vi "Read CIB.vi"(10 "COM Ref":refnum<visa-resource-name>, 11 "Cal Point":T1) -> (0 "Error Out":errorcluster, 2 "Dev Table 2":string[][](array[string]), 3 "Dev Table 1":string[][](array[string]))   [LabVIEW 2013]
uses:
  Type Defs/Cal Point Type Def.ctl
  RS485/Port Config.ctl
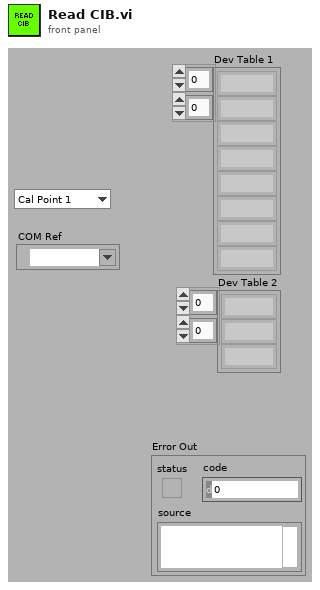
[diagram p1: front panel]
types:
  T1 = typedef "Cal Point Type Def.ctl" = enum16{"Cal Point 1", "Cal Point 2", "Cal Point 3", "Cal Point 4", "Cal Point 5", "Cal Point 6", "Cal Point 7"}
  T2 = typedef "Port Config.ctl" = cluster{"VISA resource name":refnum<visa-resource-name>, "baud rate":u32, "data bits (8)":u16, "parity (0:none)":enum16{"None", "Odd", "Even", "Mark", "Space"}, "stop bits (10: 1 bit)":u16, "flow control (0:none)":u16, "timeout (2sec)":u32}
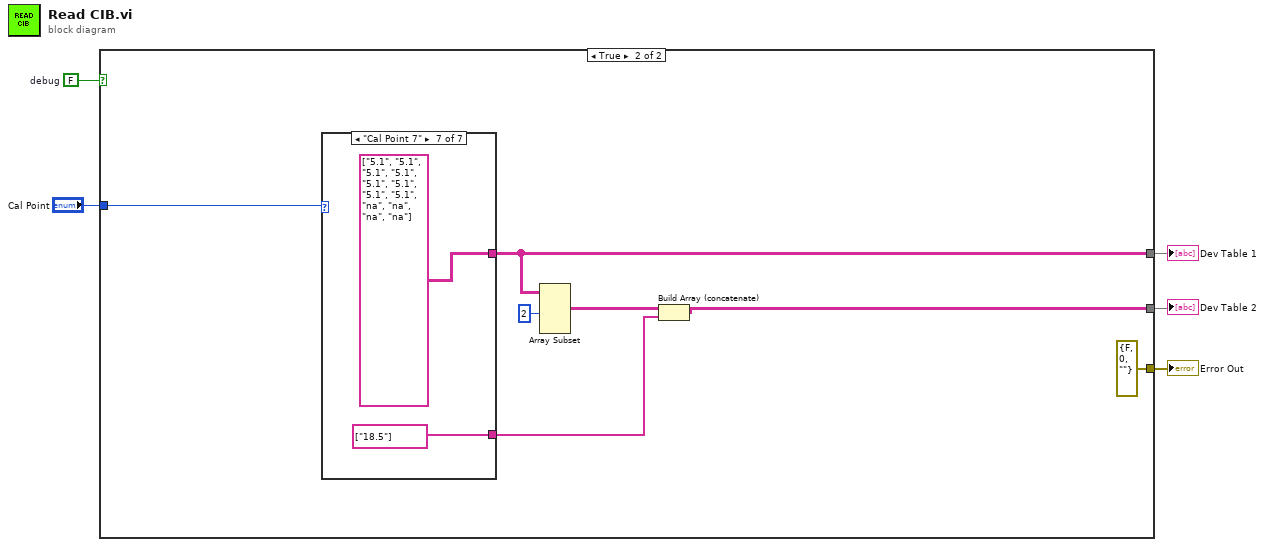
[diagram p0: block diagram]
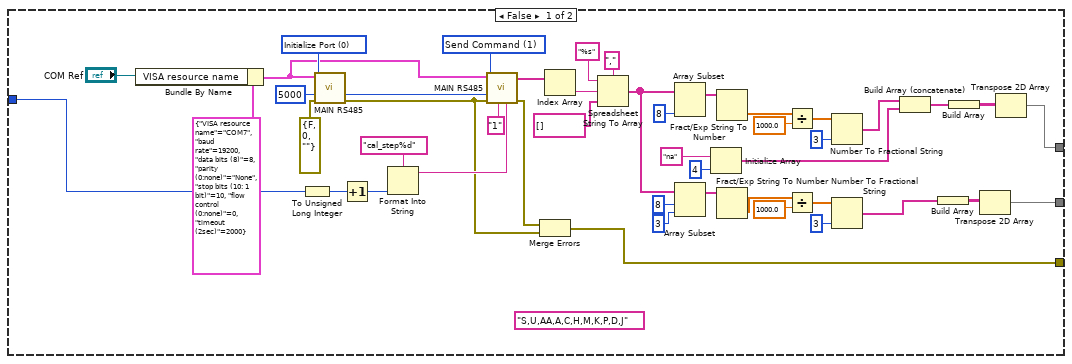
[diagram p2: hidden frame]
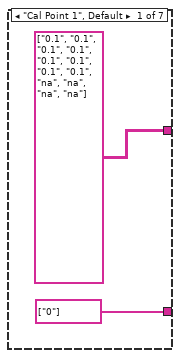
[diagram p3: hidden frame]
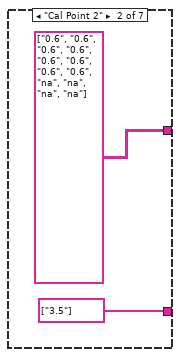
[diagram p4: hidden frame]
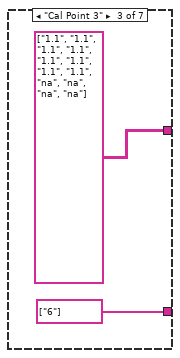
[diagram p5: hidden frame]
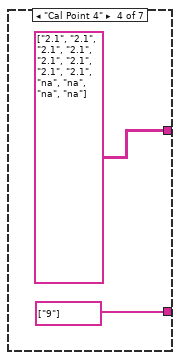
[diagram p6: hidden frame]
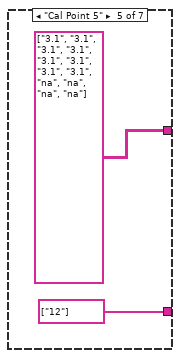
[diagram p7: hidden frame]
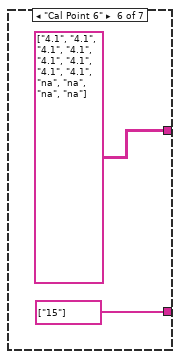
[diagram p8: hidden frame]
diagram:
  w2 = FALSE  # debug
  n1 = case shown="True" w2 {
    tunnel: "Cal Point" -> [w45 w57]
    tunnel: [w31 w56] -> w4
    tunnel: [w26 w51] -> w3
    tunnel: [w22 errorcluster {"status"=FALSE, "code"=0, "source"=""} ("Error Out")] -> w1
    frame False {
      (unwired) "S,U,AA,A,C,H,M,K,P,D,J" ("format string")
      w47 = u16 1 items=["Initialize Port", "Send Command", "Get Commands"] ("RS485 Operation")
      w18 = u32 5000 ("Timeout (ms)")
      w48 = u16 0 items=["Initialize Port", "Send Command", "Get Commands"] ("RS485 Operation")
      n2 = Bundle By Name(cluster=T2 {"VISA resource name"="COM7", "baud rate"=19200, "data bits (8)"=8, "parity (0:none)"=enum."None", "stop bits (10: 1 bit)"=10, "flow control (0:none)"=0, "timeout (2sec)"=2000} ("PortConfig"), "VISA resource name"="COM Ref") -> (w19:T2)
      n3 = To Unsigned Long Integer(number=w45) -> (unsigned 32bit integer=w44:u32)
      n4 = call "MAIN RS485.vi"("Error In"=errorcluster {"status"=FALSE, "code"=0, "source"=""}, "Timeout (ms)"=w18, "RS485 Operation"=w48, "PortConfig"=w19) -> ("Error Out"=w23:errorcluster)  [unwired: 6 in, 1 out]
      n5 = Increment(x=w44) -> (x+1=w43:u32)
      n6 = Format Into String(format string="cal_step%d" ("CIB address"), w43) -> (resulting string=w42:string)  [unwired: 2 in, 1 out]
      n7 = call "MAIN RS485.vi"("message"=w42, "CIB address"="1", "Error In"=w23, "Timeout (ms)"=w18, "RS485 Operation"=w47, "PortConfig"=w19) -> ("Error Out"=w24:errorcluster, "Return String[]"=w25:string[])  [unwired: 4 in]
      n8 = Merge Errors(w24, w23) -> (w22:errorcluster)
      n9 = Index Array(array=w25) -> (element=w20:string)  [unwired: 1 in]
      n10 = Spreadsheet String To Array(delimiter (Tab)=",", format string="%s", spreadsheet string=w20, array type (2D Dbl)=string[] []) -> (array=w29:string[])
      n11 = Array Subset(array=w29, length=8) -> (w17:string[])  [unwired: 1 in]
      n12 = Array Subset(array=w29, index=8, length=3) -> (w7:string[])
      n13 = Initialize Array("na" ("format string"), 4 ("dimension size")) -> (w34:string[])
      n14 = Fract/Exp String To Number(string=w17) -> (number=w16:dbl[])  [unwired: 3 in, 1 out]
      n15 = Fract/Exp String To Number(string=w7) -> (number=w6:dbl[])  [unwired: 3 in, 1 out]
      n16 = Divide(x=w16, y=1000.0) -> (x/y=w14:dbl[])
      n17 = Divide(x=w6, y=1000.0) -> (x/y=w10:dbl[])
      n18 = Number To Fractional String(number=w14, precision (6)=i16 3) -> (F-format string=w12:string[])  [unwired: 2 in]
      n19 = Number To Fractional String(number=w10, precision (6)=i16 3) -> (F-format string=w8:string[])  [unwired: 2 in]
      n20 = Build Array (concatenate)(w12, w34) -> (w33:string[])
      n21 = Build Array(w8) -> (w27:string[][])
      n22 = Build Array(w33) -> (w32:string[][])
      n23 = Transpose 2D Array(2D array=w27) -> (transposed array=w26:string[][])
      n24 = Transpose 2D Array(2D array=w32) -> (transposed array=w31:string[][])
    }
    frame True {
      n25 = case shown="\"Cal Point 7\"" w57 {
        tunnel: [string[][] [["0.1"], ["0.1"], ["0.1"], ["0.1"], ["0.1"], ["0.1"], ["0.1"], ["0.1"], ["na"], ["na"], ["na"], ["na"]] string[][] [["0.6"], ["0.6"], ["0.6"], ["0.6"], ["0.6"], ["0.6"], ["0.6"], ["0.6"], ["na"], ["na"], ["na"], ["na"]] string[][] [["1.1"], ["1.1"], ["1.1"], ["1.1"], ["1.1"], ["1.1"], ["1.1"], ["1.1"], ["na"], ["na"], ["na"], ["na"]] string[][] [["2.1"], ["2.1"], ["2.1"], ["2.1"], ["2.1"], ["2.1"], ["2.1"], ["2.1"], ["na"], ["na"], ["na"], ["na"]] string[][] [["3.1"], ["3.1"], ["3.1"], ["3.1"], ["3.1"], ["3.1"], ["3.1"], ["3.1"], ["na"], ["na"], ["na"], ["na"]] string[][] [["4.1"], ["4.1"], ["4.1"], ["4.1"], ["4.1"], ["4.1"], ["4.1"], ["4.1"], ["na"], ["na"], ["na"], ["na"]] string[][] [["5.1"], ["5.1"], ["5.1"], ["5.1"], ["5.1"], ["5.1"], ["5.1"], ["5.1"], ["na"], ["na"], ["na"], ["na"]]] -> w56
        tunnel: [string[] ["0"] string[] ["3.5"] string[] ["6"] string[] ["9"] string[] ["12"] string[] ["15"] string[] ["18.5"]] -> w52
        frame "Cal Point 1", Default {
        }
        frame "Cal Point 2" {
        }
        frame "Cal Point 3" {
        }
        frame "Cal Point 4" {
        }
        frame "Cal Point 5" {
        }
        frame "Cal Point 6" {
        }
        frame "Cal Point 7" {
        }
      }
      n26 = Array Subset(array=w56, length (row)=2 ("length")) -> (w53:string[][])  [unwired: 3 in]
      n27 = Build Array (concatenate)(w53, w52) -> (w51:string[][])
    }
  }
  "Dev Table 1" <- w4
  "Dev Table 2" <- w3
  "Error Out" <- w1
